vi "Tab_006_PH.vi"() -> ()   [LabVIEW 2021]
panel:
  out "Array 2":dbl[][](array[numeric])
  out "indeks j":i32=4
  out "indeks i":i32=2
  in  "Array":dbl[][](array[numeric])=[[11.0, 12.0, 13.0, 14.0, 15.0], [21.0, 22.0, 23.0, 24.0, 25.0], [31.0, 32.0, 33.0, 34.0, 35.0]]
  # "indeks i = 0, 1,2,"
  # "indeks j =0,1,2,3,4,"
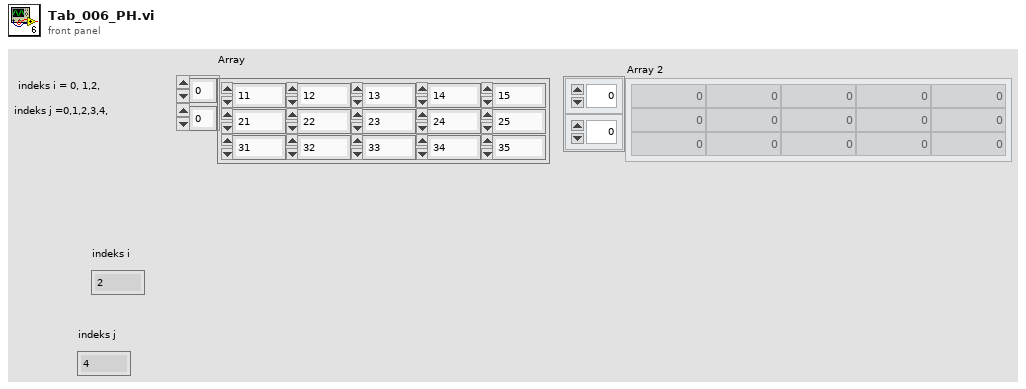
[diagram p1: front panel]
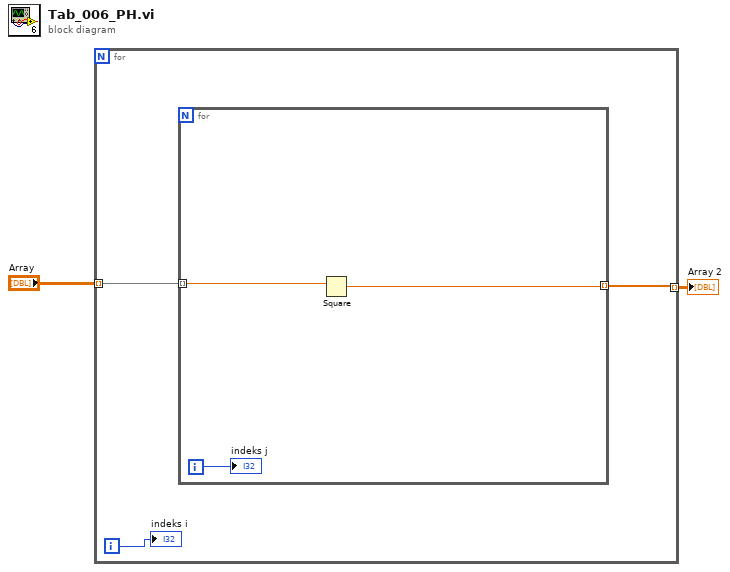
[diagram p0: block diagram]
diagram:
  n1 = for {
    tunnel: "Array" -> [w4] mode=indexing
    tunnel: [w3] -> w1 mode=indexing
    i -> [w5]
    n2 = for {
      tunnel: w4 -> [w7] mode=indexing
      tunnel: [w6] -> w3 mode=indexing
      i -> [w8]
      n3 = Square(x=w7) -> (x^2=w6:dbl)
      "indeks j" <- w8
    }
    "indeks i" <- w5
  }
  "Array 2" <- w1
